vi "Actor Core.vi"(8 "error in":errorcluster, 11 "DIMDemoServer in":refnum<class "DIMDemoServer.lvclass">) -> (0 "error out":errorcluster, 3 "Actor out":refnum<class "Actor.lvclass">)   [LabVIEW 2012, in "DimActorDemo.lvlib" / "DIMDemoServer.lvclass"]
doc: "(<B>Filename</B>: Actor Framework.lvlib:Actor.lvclass:Actor Core.vi)\n\nReceives messages to the actor, reacts to them, and initiates any error handling that may shut the actor down.\n\nDescendant classes may override this VI to append parallel tasks for the actor to complete while it handles messages. Overrides use the Call Parent Method node."
uses:
  DIMDemoServer.lvclass
  <vilib>/ActorFramework/Actor/Actor.lvclass
  DIMActor/DIMActor/DIMActor.lvclass/DIMActor.ctl
  DIMActor/DIMActor/DIMActor.lvclass
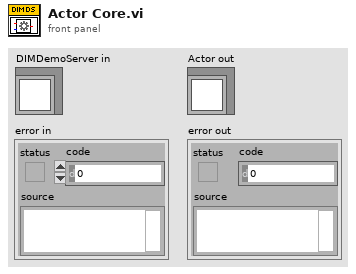
[diagram p1: front panel]
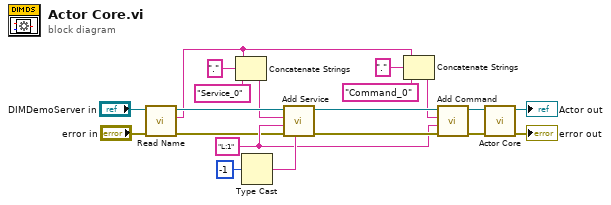
[diagram p0: block diagram]
diagram:
  w12 = "L:1" ("Type Descriptor")
  n1 = call "Read Name.vi"("error in (no error)"="error in", "DIMActor in"="DIMDemoServer in") -> ("error out"=w8:errorcluster, "Name"=w3:string, "DIMActor out"=w10:refnum<class "DIMDemoServer.lvclass">)  [unwired: 7 in]
  n2 = Concatenate Strings(w3, "." ("string"), "Service_0" ("Service Name")) -> (w5:string)
  n3 = Type Cast(x=-1) -> (*(type *) &x=w14:string)  [unwired: 1 in]
  n4 = call "Add Service.vi"("Data"=w14, "error in (no error)"=w8, "Type Descriptor"=w12, "Service Name"=w5, "DIMActor in"=w10) -> ("error out"=w17:errorcluster, "DIMActor out"=w18:refnum<class "DIMDemoServer.lvclass">)  [unwired: 5 in]
  n5 = Concatenate Strings(w3, "." ("string"), "Command_0" ("Command Name")) -> (w1:string)
  n6 = call "Add Command.vi"("error in (no error)"=w17, "Type Descriptor"=w12, "Command Name"=w1, "DIMActor in"=w18) -> ("error out"=w16:errorcluster, "DIMActor out"=w15:refnum<class "DIMDemoServer.lvclass">)  [unwired: 6 in]
  n7 = call-parent "Actor Core.vi"("error in"=w16, "DIMActor in"=w15) -> ("error out"=→"error out":errorcluster, "Actor out"=→"Actor out":refnum<class "Actor.lvclass">)  [unwired: 8 in]
